vi "PVCAM_DDIGetVer.vi"(8 "error in (no error)":errorcluster) -> (0 "error out":errorcluster, 2 "return type":i16, 3 "version out":u16)   [LabVIEW 2021]
uses:
  Windows/System32/pvcam64.dll
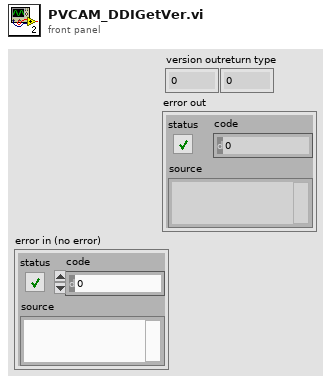
[diagram p1: front panel]
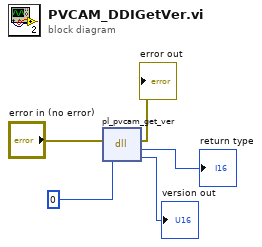
[diagram p0: block diagram]
diagram:
  n1 = dll-call lib="C:/Windows/System32/pvcam64.dll" fn="pl_pvcam_get_ver"(error in="error in (no error)", "version"=u16 0) -> (error out=→"error out":errorcluster, "return type"=→"return type":i16, "version"=→"version out":u16)  [unwired: 2 in, 1 out]
